vi "BodeMagnitudePlot.vi"() -> ()   [LabVIEW 2014]
uses:
  <vilib>/imath/engines/lvmath2/RunTimeEngine/Managers/WorkSpace/UID Generator.vi
  <vilib>/imath/engines/lvmath2/RunTimeEngine/RunTimeType/NIMS_RunTimeType_From StrictType (excl LVString).vi
  <instcachedir>/0/NIMS_RunTimeType_From StrictType (excl LVString)_15A5391EEA9C4AACB9955AC755B83D29.lvgen/NIMS_RunTimeType_From StrictType (excl LVString)_15A5391EEA9C4AACB9955AC755B83D29_000.vi
  <vilib>/imath/engines/lvmath2/RunTimeEngine/LocalVariableDefStatement/MC_LocalVariableDefStatement_Display.vi
  <vilib>/imath/engines/lvmath2/RunTimeEngine/Managers/SymbolTable/Clear UID.vi
  <vilib>/imath/engines/lvmath2/RunTimeEngine/NodeEndStatement/NIMS_NodeEndStatement_Output.vi
  <instcachedir>/0/NIMS_NodeEndStatement_Output_53EC0D466D134D7ABD903AC30B43404B.lvgen/NIMS_NodeEndStatement_Output_53EC0D466D134D7ABD903AC30B43404B_000.vi
  <vilib>/imath/engines/lvmath2/RunTimeEngine/ErrorHandling/NIMS_Finalize Error.vi
  <vilib>/Analysis/NI_AALPro.lvlib
  <vilib>/imath/engines/lvmath2/RunTimeEngine/Managers/SymbolTable/NIMS_WorkSpace.lvlib
panel:
  out "XY Graph":cluster{"f":dbl[], dbl[]}(graph)={"f"=[10.0, 35.0, 60.0, 85.0, 110.0, 135.0, 160.0, 185.0, 210.0, 235.0, 260.0, 285.0, 310.0, 335.0, 360.0, 385.0, 410.0, 435.0, 460.0, 485.0, 510.0, 535.0, 560.0, 585.0, 610.0, 635.0, 660.0, 685.0, 710.0, 735.0, 760.0, 785.0, 810.0, 835.0, 860.0, 885.0, 910.0, 935.0, 960.0, 985.0, 1010.0, 1035.0, 1060.0, 1085.0, 1110.0, 1135.0, 1160.0, 1185.0, 1210.0, 1235.0, 1260.0, 1285.0, 1310.0, 1335.0, 1360.0, 1385.0, 1410.0, 1435.0, 1460.0, 1485.0, 1510.0, 1535.0, 1560.0, 1585.0, 1610.0, 1635.0, 1660.0, 1685.0, 1710.0, 1735.0, 1760.0, 1785.0, 1810.0, 1835.0, 1860.0, 1885.0, 1910.0, 1935.0, 1960.0, 1985.0, 2010.0], [-3.014865581126763, -3.0141454856299585, -3.0596718785653665, -3.1518645231854125, -3.2883110150855313, -3.465286850867381, -3.6774755266054093, -3.919198946954811, -4.1861772143729015, -4.472738895731544, -4.773602649356024, -5.085457934257826, -5.404662819647374, -5.728005471380396, -6.053594391060379, -6.378566129219944, -6.70152204142169, -7.02092018871536, -7.337276782590143, -7.648521013505601, -7.954270670488076, -8.254863831824625, -8.549106968030815, -8.837788373895329, -9.120480365190497, -9.396510705562923, -9.66734200802653, -9.931734345937006, -10.18983984776295, -10.442230508254848, -10.689054029817488, -10.929882415998733, -11.16661675913975, -11.397496954625971, -11.622787199687165, -11.843919715827598, -12.060542650380988, -12.271987299314173, -12.479689741928393, -12.68197049031935, -12.882346718411856, -13.077041023193097, -13.267956728230196, -13.455825771625694, -13.63968563727475, -13.820479791004548, -13.99783026261212, -14.171856944321174, -14.342456998010501, -14.510395375662654, -14.674761050325916, -14.837973981204001, -14.996754307621746, -15.154062034252592, -15.3073586148355, -15.45869497536582, -15.608906121388289, -15.754380292707125, -15.90030680250812, -16.042753003259286, -16.183734849462898, -16.32228135625192, -16.456408435783867, -16.59002246221843, -16.721666316311897, -16.85280149127103, -16.982532188564534, -17.108770804714887, -17.23269608883364, -17.356063506596758, -17.477916324427476, -17.59800247537126, -17.715852589325657, -17.834089140147455, -17.949115114246435, -18.06523758191328, -18.17473694041105, -18.2875428685297, -18.395473834183246, -18.506489579175597, -18.613909722657425]}
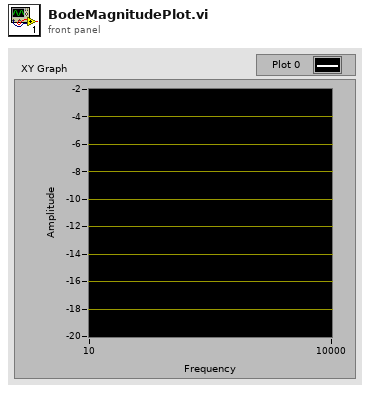
[diagram p1: front panel]
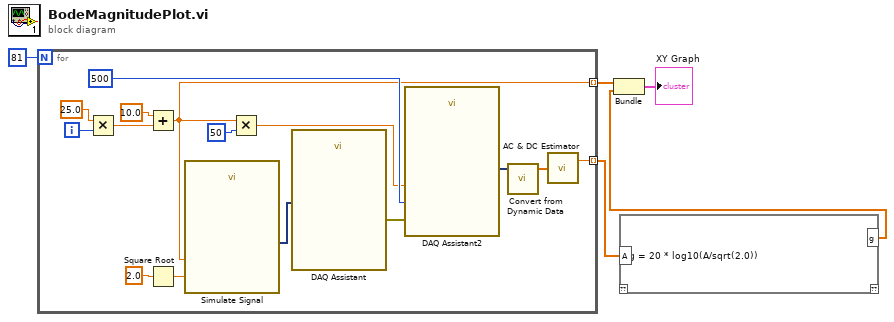
[diagram p0: block diagram]
diagram:
  n1 = for {
    N: 81 -> [_]
    tunnel: [w7] -> w2 mode=indexing
    tunnel: [w6] -> w4 mode=indexing
    i -> [w10]
    n2 = Multiply(x=25.0, y=w10) -> (x*y=w9:dbl)
    n3 = Add(x=10.0, y=w9) -> (x+y=w6:dbl)
    n4 = Square Root(x=2.0) -> (sqrt(x)=w20:dbl)
    n5 = call "Simulate Signal"("Frequency"=w6, "Amplitude"=w20) -> ("Sine"=w19:dynamicdata)  [unwired: 12 in, 1 out]
    n6 = Multiply(x=w6, y=50) -> (x*y=w15:dbl)
    n7 = call "DAQ Assistant"("data"=w19) -> ("error out"=w18:errorcluster)  [unwired: 16 in, 2 out]
    n8 = call "DAQ Assistant2"("rate"=w15, "number of samples"=500, "error in"=w18) -> ("data"=w14:dynamicdata)  [unwired: 14 in, 2 out]
    n9 = call "Convert from Dynamic Data"("Dynamic Data Type"=w14) -> ("Array"=w13:dbl[])  [unwired: 3 in]
    n10 = call <vilib>:"AC & DC Estimator.vi"("Signal (V)"=w13) -> ("AC estimate (Vrms)"=w7:dbl)  [unwired: 1 out]
  }
  n11 = mathscript code="g = 20 * log10(A/sqrt(2.0))"("A"=w2) -> ("g"=w1:cdb[])  [unwired: 1 in, 1 out]
  n12 = Bundle(w4, "g"=w1) -> (→"XY Graph":cluster{dbl[], "g":cdb[]})  [unwired: 1 in]
